vi "Auto 8.vi"(8 "Error In":errorcluster) -> (0 "Error Out":errorcluster)   [LabVIEW 2014]
uses:
  <vilib>/Rock Robotics/Network Tables/SD Read Boolean.vi
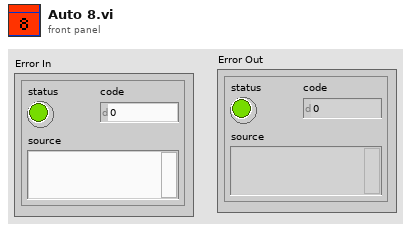
[diagram p1: front panel]
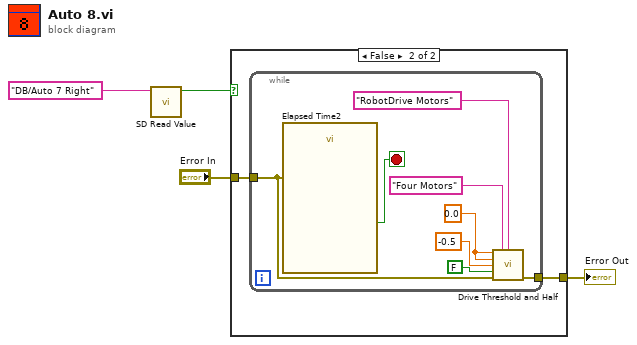
[diagram p0: block diagram]
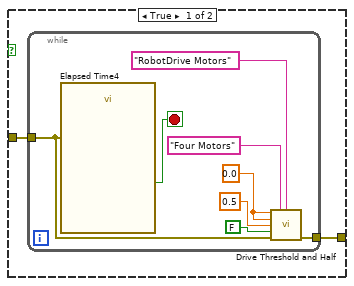
[diagram p2: hidden frame]
diagram:
  n1 = call-poly <vilib>:"SD Read Value.vi"("Name"="DB/Auto 7 Right") -> ("Boolean"=w3:bool)  [unwired: 8 in, 2 out]
  n2 = case shown="False" w3 {
    tunnel: "Error In" -> [w6 w16]
    tunnel: [w5 w15] -> w1
    frame True {
      n3 = while {
        tunnel: w6 -> [w7]
        tunnel: [w11] -> w5
        stop <- w8 stop-if-true
        w10 = 0.0 ("Arm Value")
        n4 = call "Elapsed Time4"("error in (no error)"=w7) -> ("Time has Elapsed"=w8:bool)  [unwired: 11 in, 7 out]
        n5 = call "Drive Threshold and Half.vi"("X In"=w10, "Drive refnum name"="Four Motors" ("refnum name"), "Send to DB Name"="RobotDrive Motors" ("Name"), "Y In"=w10, "R In"=0.5 ("X In"), "Speed Toggle"=FALSE ("Grabber Open/Close"), "Error In"=w7) -> ("Error Out"=w11:errorcluster)  [unwired: 8 in]
      }
    }
    frame False {
      n6 = while {
        tunnel: w16 -> [w17]
        tunnel: [w19] -> w15
        stop <- w18 stop-if-true
        w21 = 0.0 ("Arm Value")
        n7 = call "Elapsed Time2"("error in (no error)"=w17) -> ("Time has Elapsed"=w18:bool)  [unwired: 11 in, 7 out]
        n8 = call "Drive Threshold and Half.vi"("X In"=w21, "Drive refnum name"="Four Motors" ("refnum name"), "Send to DB Name"="RobotDrive Motors" ("Name"), "Y In"=w21, "R In"=-0.5 ("X In"), "Speed Toggle"=FALSE ("Grabber Open/Close"), "Error In"=w17) -> ("Error Out"=w19:errorcluster)  [unwired: 8 in]
      }
    }
  }
  "Error Out" <- w1
